vi "SubVI_ProcessTitle.vi"(11 "Title":string[](array[string])) -> (3 "Array":T1[](array[typedef]))   [LabVIEW 2011]
uses:
  Data File Processing UI_ChannelSet.ctl
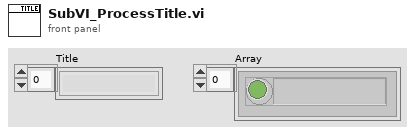
[diagram p1: front panel]
types:
  T1 = typedef "Data File Processing UI_ChannelSet.ctl" = cluster{"Select":bool, "Channel":string}
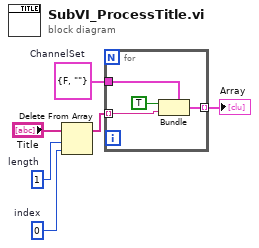
[diagram p0: block diagram]
diagram:
  w1 = 1  # length
  w2 = 0  # index
  w5 = T1 {"Select"=FALSE, "Channel"=""}  # ChannelSet
  n1 = Delete From Array(array="Title", length=w1, index=w2) -> (array with subset deleted=w3:string[])  [unwired: 1 out]
  n2 = for {
    tunnel: w3 -> [w9] mode=indexing
    tunnel: w5 -> [w8]
    tunnel: [w7] -> w6 mode=indexing
    n3 = Bundle(cluster=w8, "Select"=TRUE, "Channel"=w9) -> (w7:T1)
  }
  "Array" <- w6
